vi "Clusterwitharraypath.vi"(1 "Cluster In":cluster{"Array In":path[], "Path":path}, 2 "Path To Append":path) -> (0 "Cluster Out":cluster{"Array Out":path[], "Path":path})   [LabVIEW 2011]
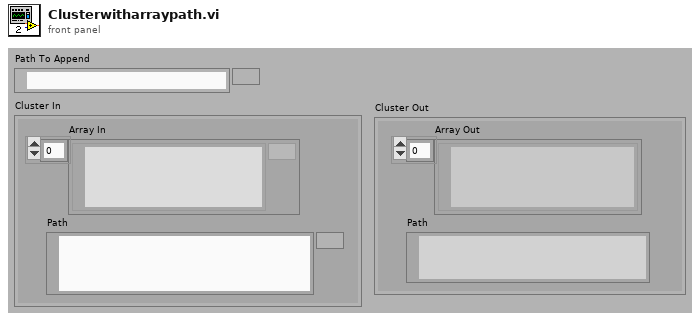
[diagram p1: front panel]
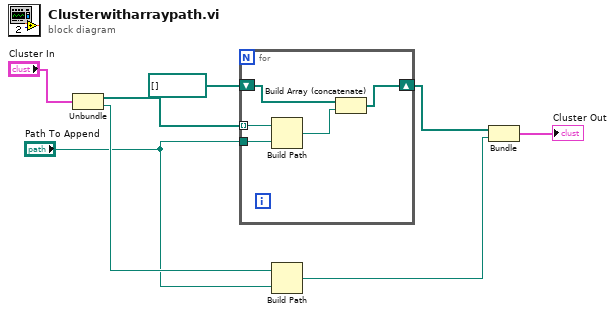
[diagram p0: block diagram]
diagram:
  n1 = Unbundle("Cluster In") -> ("Array In"=w6:path[], "Path"=w3:path)
  n2 = for {
    tunnel: w6 -> [w10] mode=indexing
    shift-right: [w12] -> w4
    shift-left: path[] [] -> [w13]
    tunnel: "Path To Append" -> [w9]
    n3 = Build Path(base path=w10, name or relative path=w9) -> (appended path=w11:path)
    n4 = Build Array (concatenate)(w13, w11) -> (w12:path[])
  }
  n5 = Build Path(base path=w3, name or relative path="Path To Append") -> (appended path=w1:path)
  n6 = Bundle(w4, "appended path"=w1) -> (→"Cluster Out":cluster{path[], "appended path":path})  [unwired: 1 out]
